vi "MultiChannelType_2D-Array-I16.vi"(9 "error in":errorcluster, 11 "Array in":i16[][](array[numeric])) -> (1 "error out":errorcluster, 2 "MultiChannelType":u64, 3 "Array out":i16[][](array[numeric]))   [LabVIEW 2020, in "OpenLvVision_OpenCv.lvlib"]
uses:
  OpenLvVision_OpenCv.lvlib
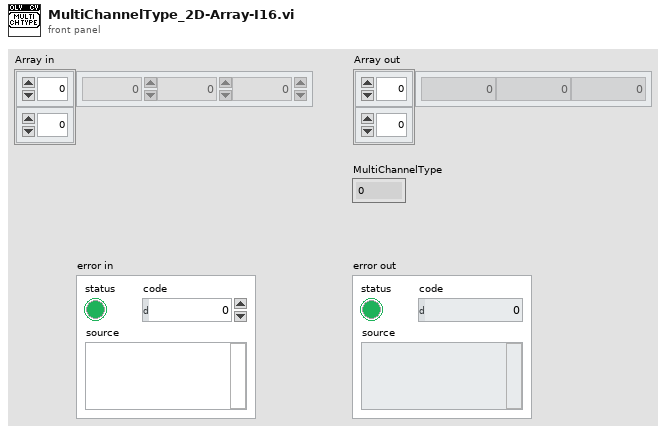
[diagram p1: front panel]
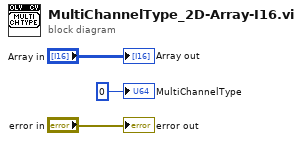
[diagram p0: block diagram]
diagram:
  "error out" <- "error in"
  "Array out" <- "Array in"
  "MultiChannelType" <- u64 0
